vi "DefaultFromIni.vi"(8 "error in (no error)":errorcluster, 11 "ChromaAcLoad":refnum<class "ChromaAcLoad.lvclass">) -> (0 "error out":errorcluster, 3 "ChromaAcLoad":refnum<class "ChromaAcLoad.lvclass">)   [LabVIEW 2018, in "AcPwrPlugins.lvlib" / "ChromaAcLoad.lvclass"]
uses:
  ChromaAcLoad.lvclass
  C:/Program Files (x86)/National Instruments/LabVIEW 2018/user.lib/NIST/BaseClasses/BasePlugin_class/BasePlugin.lvclass
  TypeDefs/Load.ctl
  TypeDefs/LoadSettings.ctl
  TypeDefs/LC.ctl
  TypeDefs/LoadModes.ctl
  <userlib>/NIST/BaseClasses/BasePlugin_class/BasePlugin.lvclass/BasePlugin.ctl
  ChromaAcLoad.lvclass/ChromaAcLoad.ctl
  <userlib>/NIST/BaseClasses/BasePlugin_class/Accessors/Read PluginIniFilePath.vi
  Accessors/Write Loads.vi
  AcPwrBaseClass/AcPwrBase.lvclass
  <vilib>/Utility/config.llb/NI_LVConfig.lvlib
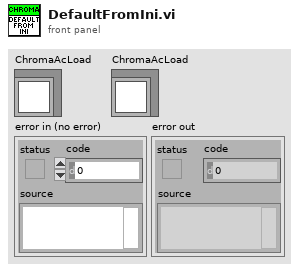
[diagram p1: front panel]
types:
  T1 = typedef "AcPwrPlugins.lvlib/ChromaAcLoad.lvclass/Load.ctl" = cluster{"AC/DC":bool, "Resistance":dbl, "LoadSettings":T2, "Wave":enum16{""}, "LineSync":bool, "LoadShortCircuited":bool, "LC":T3, "Timing":cluster{"TimingOn":enum16{""}, "Hours":u32, "Minutes":u32, "Seconds":dbl, "CutoffVoltage":dbl}, "Slew":cluster{"RiseSlewRate":i32, "FallSlewRate":i32}, "Mode":T4}
  T2 = typedef "AcPwrPlugins.lvlib/ChromaAcLoad.lvclass/LoadSettings.ctl" = cluster{"CrestFactor":dbl, "PowerFactor":dbl, "PowerLoading":dbl, "IpeakMax":dbl, "Priority":enum16{"CF Only", "PF Only", "Both (CF)", "Both (PF)"}, "ILoad":dbl}
  T3 = typedef "AcPwrPlugins.lvlib/ChromaAcLoad.lvclass/LC.ctl" = cluster{"C (uF)":i32, "LS (uH)":i32, "RL (Ohm)":dbl, "RS (Ohm)":dbl}
  T4 = typedef "AcPwrPlugins.lvlib/ChromaAcLoad.lvclass/LoadModes.ctl" = enum16{"CC", "CP", "CV", "CR", "RLC", "RLC CP", "Inrush", "Rectified"}
  T5 = typedef "NI_LVConfig.lvlib/Config Data RefNum.ctl" = refnum<k1>
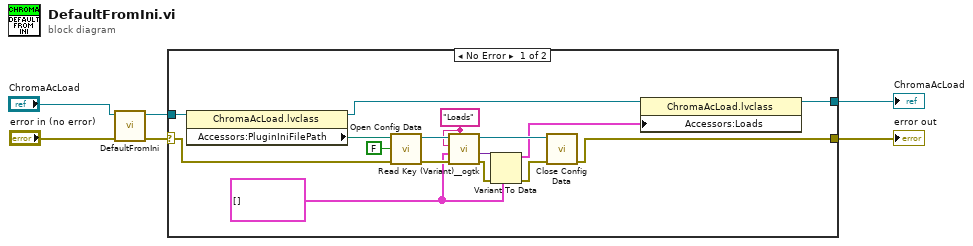
[diagram p0: block diagram]
diagram:
  n1 = call-parent "DefaultFromIni.vi"("error in (no error)"="error in (no error)", "AcPwrBase"="ChromaAcLoad") -> ("error out"=w4:errorcluster, "AcPwrBase"=w3:refnum<class "ChromaAcLoad.lvclass">)  [unwired: 8 in]
  n2 = case shown="No Error" w4 {
    selector: w4 -> [w19 w23]
    tunnel: w3 -> [w22 w24]
    tunnel: [w13 w24] -> w2
    tunnel: [w10 w23] -> w1
    frame No Error {
      w8 = T1[] []
      w9 = "Loads" ("section")
      n3 = property class="ChromaAcLoad.lvclass"(reference=w22) -> (reference out=w14:refnum<class "ChromaAcLoad.lvclass">, "Accessors:PluginIniFilePath"=w21:path)  [unwired: 1 in, 1 out]
      n4 = call <vilib>:"Open Config Data.vi"("error in (no error)"=w19, "create file if necessary (T)"=FALSE, "configuration file path"=w21) -> ("error out"=w17:errorcluster, "refnum"=w18:T5)  [unwired: 6 in, 1 out]
      n5 = call <userlib>:"Read Key (Variant)__ogtk.vi"("section"=w9, "error in (no error)"=w17, "type"=w8, "key (optional)"=w9, "refnum"=w18) -> ("error out"=w15:errorcluster, "key-value"=w16:variant, "refnum out"=w12:T5)  [unwired: 3 in, 1 out]
      n6 = Variant To Data(error in=w15, type=w8, Variant=w16) -> (data=w7:T1[], error out=w11:errorcluster)
      n7 = call <vilib>:"Close Config Data.vi"("error in (no error)"=w11, "refnum"=w12) -> ("error out"=w10:errorcluster)  [unwired: 8 in, 1 out]
      n8 = property class="ChromaAcLoad.lvclass"(reference=w14, "Accessors:Loads"=w7) -> (reference out=w13:refnum<class "ChromaAcLoad.lvclass">)  [unwired: 1 in, 1 out]
    }
    frame Error {
    }
  }
  "error out" <- w1
  "ChromaAcLoad" <- w2
